vi "Get Localhost Name.vi"(8 "error in (no error)":errorcluster, 11 "Interface_Class in":refnum<class "Abstraction_Interface_Class.lvclass">) -> (0 "error out":errorcluster, 1 "PC Name":string, 3 "Interface_Class out":refnum<class "Abstraction_Interface_Class.lvclass">)   [LabVIEW 2023, in "Abstraction_Interface.lvlib" / "Abstraction_Interface_Class.lvclass"]
uses:
  Abstraction_Interface_Class.lvclass
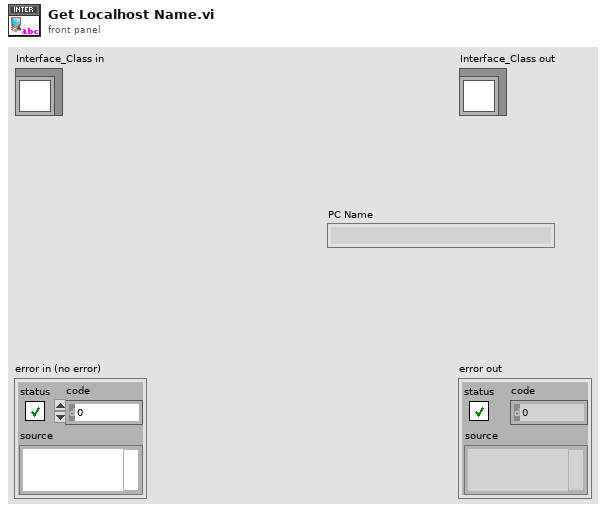
[diagram p1: front panel]
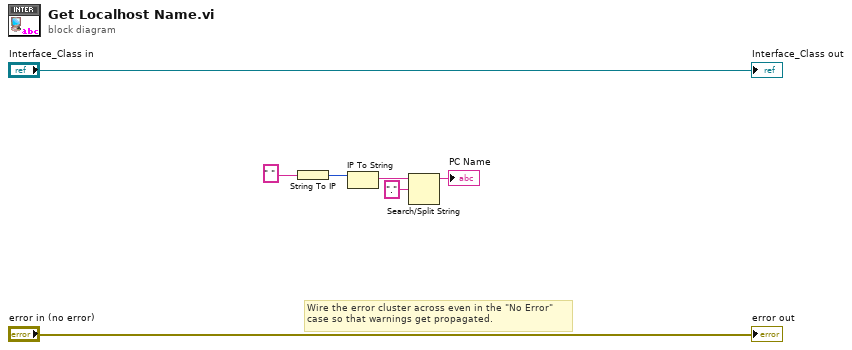
[diagram p0: block diagram]
diagram:
  # "Wire the error cluster across even in the \"No Error\"\ncase so that warnings get propagated."
  n1 = String To IP(1:" " ("name")) -> (0:w5:u32)
  n2 = IP To String(2:w5) -> (0:w4:string)  [unwired: 1 in]
  n3 = Search/Split String(string=w4, search string/char (-)=".") -> (substring before match=→"PC Name":string)  [unwired: 1 in, 2 out]
  "error out" <- "error in (no error)"
  "Interface_Class out" <- "Interface_Class in"
